vi "Map Channels.vi"(8 "error in (no error)":errorcluster, 11 "Red Pitaya Digitizer in":refnum<class "Red Pitaya Digitizer.lvclass">) -> (0 "error out":errorcluster, 3 "Red Pitaya Digitizer out":refnum<class "Red Pitaya Digitizer.lvclass">)   [LabVIEW 2024, in "Red Pitaya Digitizer.lvclass"]
uses:
  Red Pitaya Digitizer.lvclass
  Red Pitaya Digitizer.lvclass/Red Pitaya Digitizer.ctl
  RP Core/RP Instrument/RP Instrument.lvclass
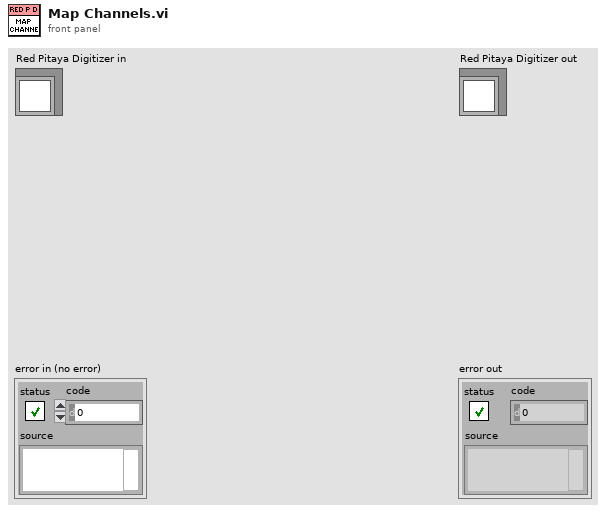
[diagram p1: front panel]
types:
  T1 = map{i32, cluster{"Module":i32, "Local channel":i32}}
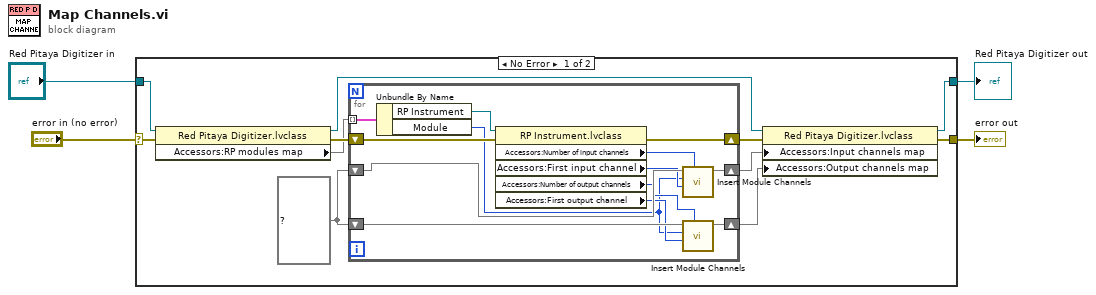
[diagram p0: block diagram]
diagram:
  n1 = case shown="No Error" "error in (no error)" {
    selector: "error in (no error)" -> [w13 w30]
    tunnel: [w11 w30] -> w3
    tunnel: [w9 w29] -> w1
    tunnel: "Red Pitaya Digitizer in" -> [w14 w29]
    frame No Error {
      w6 = T1 {} ("Channels map out")
      n2 = property class="Red Pitaya Digitizer.lvclass"(reference=w14, error in=w13) -> (reference out=w10:refnum<class "Red Pitaya Digitizer.lvclass">, error out=w15:errorcluster, "Accessors:RP modules map "=w5:map{i32, refnum<class "RP Instrument.lvclass">})
      n3 = for {
        shift-right: [w27] -> w12
        shift-left: w15 -> [w28]
        shift-right: [w25] -> w8
        shift-left: w6 -> [w26]
        shift-right: [w23] -> w7
        shift-left: w6 -> [w24]
        tunnel: w5 -> [w18] mode=indexing
        n4 = Unbundle By Name(w18) -> ("RP Instrument"=w17:refnum<class "RP Instrument.lvclass">, "Module"=w16:i32)
        n5 = property class="RP Instrument.lvclass"(reference=w17, error in=w28) -> (error out=w27:errorcluster, "Accessors:Number of input channels"=w22:i32, "Accessors:First input channel"=w21:i32, "Accessors:Number of output channels"=w20:i32, "Accessors:First output channel"=w19:i32)  [unwired: 1 out]
        n6 = call "Insert Module Channels.vi"("Number of channels"=w22, "First channel"=w21, "Module"=w16, "Channels map"=w26) -> ("Channels map out"=w25:T1)  [unwired: 7 in]
        n7 = call "Insert Module Channels.vi"("Number of channels"=w20, "First channel"=w19, "Module"=w16, "Channels map"=w24) -> ("Channels map out"=w23:T1)  [unwired: 7 in]
      }
      n8 = property class="Red Pitaya Digitizer.lvclass"(reference=w10, error in=w12, "Accessors:Input channels map"=w8, "Accessors:Output channels map"=w7) -> (reference out=w9:refnum<class "Red Pitaya Digitizer.lvclass">, error out=w11:errorcluster)
    }
    frame Error {
    }
  }
  "error out" <- w3
  "Red Pitaya Digitizer out" <- w1
